vi "Configure Ethernet.vi"(0 "VISA resource name":refnum<visa-resource-name>, 1 "Differential Input Data Source (0: Channel 1)":u16(ring) items=["Channel 1", "Channel 2", "Channel 3", "Channel 4", "Math", "Reference 1", "Reference 2", "Reference 3", "Reference 4"], 2 "Ethernet D+ Data Source (0: Channel 1)":u16(ring) items=["Channel 1", "Channel 2", "Channel 3", "Channel 4"], 5 "Bus Number (9: Bus 1)":u16(ring)=9 items=["Bus 1"=9, "Bus 2"=10], 7 "Ethernet Type (0: ENET10BASET)":u16(ring) items=["ENET10BASET", "ENET100BASETX"], 9 "Probe Type (0: Differential)":u16(ring) items=["Differential", "Single Ended"], 11 "error in (no error)":errorcluster, 12 "Ethernet D- Data Source (0: Channel 1)":u16(ring) items=["Channel 1", "Channel 2", "Channel 3", "Channel 4"], 13 "Ethernet Protocol (0: IPV 4)":u16(ring) items=["IPV 4", "Other"]) -> (4 "VISA resource name out":refnum<visa-resource-name>, 15 "error out":errorcluster)   [LabVIEW 2009, in "Tektronix DPO MSO 2000 4000 Series.lvlib"]
doc: "Configures ethernet settings for an oscilloscope. \n\n<B>Note:</B>\nThis VI only applies to DPO4034B, DPO4054B, DPO4104B, MSO4034B, MSO4054B, MSO4104B."
uses:
  <instrlib>/Tektronix DPO MSO 2000 4000 Series/Tektronix DPO MSO 2000 4000 Series.lvlib
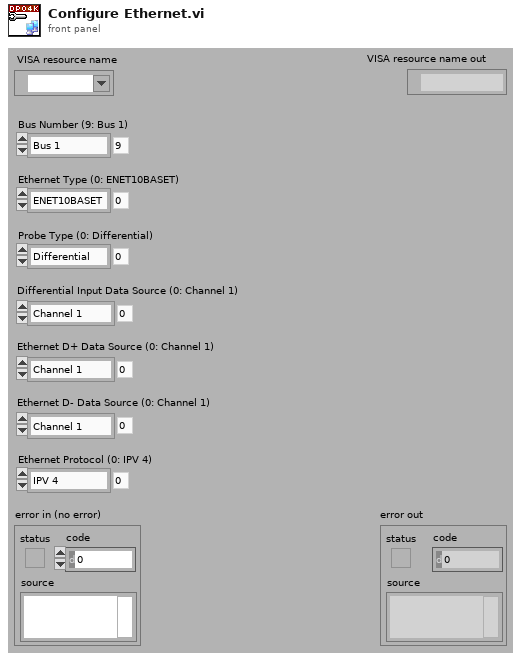
[diagram p1: front panel]
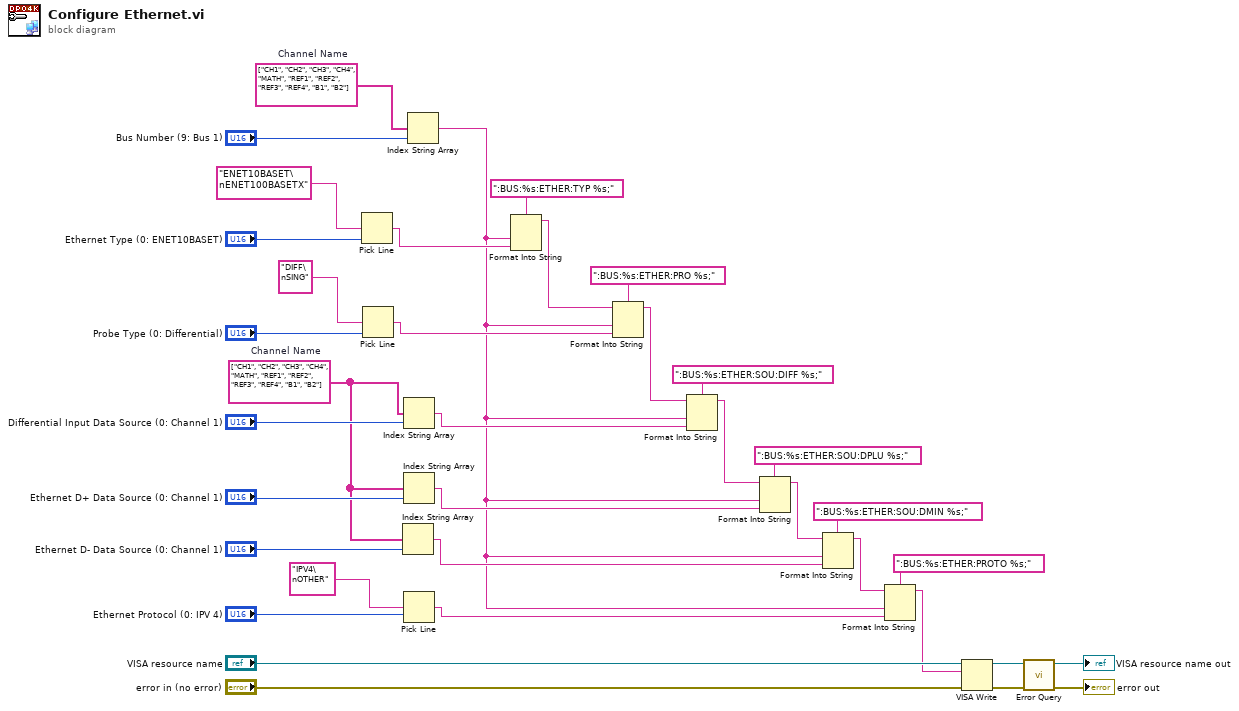
[diagram p0: block diagram]
diagram:
  w8 = string[] ["CH1", "CH2", "CH3", "CH4", "MATH", "REF1", "REF2", "REF3", "REF4", "B1", "B2"]  # Channel Name
  w31 = string[] ["CH1", "CH2", "CH3", "CH4", "MATH", "REF1", "REF2", "REF3", "REF4", "B1", "B2"]  # Channel Name
  n1 = Pick Line(multi-line string="ENET10BASET\nENET100BASETX", line index="Ethernet Type (0: ENET10BASET)") -> (output string=w26:string)  [unwired: 1 in]
  n2 = Pick Line(multi-line string="DIFF\nSING", line index="Probe Type (0: Differential)") -> (output string=w22:string)  [unwired: 1 in]
  n3 = Index String Array(1:"Ethernet D- Data Source (0: Channel 1)", 2:w8) -> (0:w13:string)  [unwired: 1 in]
  n4 = Index String Array(1:"Differential Input Data Source (0: Channel 1)", 2:w8) -> (0:w18:string)  [unwired: 1 in]
  n5 = Index String Array(1:"Ethernet D+ Data Source (0: Channel 1)", 2:w8) -> (0:w14:string)  [unwired: 1 in]
  n6 = Pick Line(multi-line string="IPV4\nOTHER", line index="Ethernet Protocol (0: IPV 4)") -> (output string=w6:string)  [unwired: 1 in]
  n7 = Index String Array(1:"Bus Number (9: Bus 1)", 2:w31) -> (0:w10:string)  [unwired: 1 in]
  n8 = Format Into String(format string=":BUS:%s:ETHER:TYP %s;", w10, w26) -> (resulting string=w5:string)  [unwired: 2 in, 1 out]
  n9 = Format Into String(format string=":BUS:%s:ETHER:PRO %s;", initial string=w5, w10, w22) -> (resulting string=w19:string)  [unwired: 1 in, 1 out]
  n10 = Format Into String(format string=":BUS:%s:ETHER:SOU:DIFF %s;", initial string=w19, w10, w18) -> (resulting string=w4:string)  [unwired: 1 in, 1 out]
  n11 = Format Into String(format string=":BUS:%s:ETHER:SOU:DPLU %s;", initial string=w4, w10, w14) -> (resulting string=w3:string)  [unwired: 1 in, 1 out]
  n12 = Format Into String(format string=":BUS:%s:ETHER:SOU:DMIN %s;", initial string=w3, w10, w13) -> (resulting string=w1:string)  [unwired: 1 in, 1 out]
  n13 = Format Into String(format string=":BUS:%s:ETHER:PROTO %s;", initial string=w1, w10, w6) -> (resulting string=w2:string)  [unwired: 1 in, 1 out]
  n14 = VISA Write(VISA resource name="VISA resource name", write buffer=w2, error in (no error)="error in (no error)") -> (VISA resource name out=w35:refnum<visa-resource-name>, error out=w34:errorcluster)  [unwired: 1 out]
  n15 = call <instrlib>:"Error Query.vi"("error in (no error)"=w34, "VISA resource name"=w35) -> ("error out"=→"error out":errorcluster, "VISA resource name out"=→"VISA resource name out":refnum<visa-resource-name>)  [unwired: 6 in, 2 out]
